vi "cRIO IO Simulation.vi"() -> ()   [LabVIEW 2024, in "cRIO1.lvlib"]
doc: "Simulates a PID controller."
uses:
  cRIO1.lvlib
  PID - Data.ctl
panel:
  out "error out":errorcluster
  out "output chart":dbl(graph)
  in  "Stop":bool
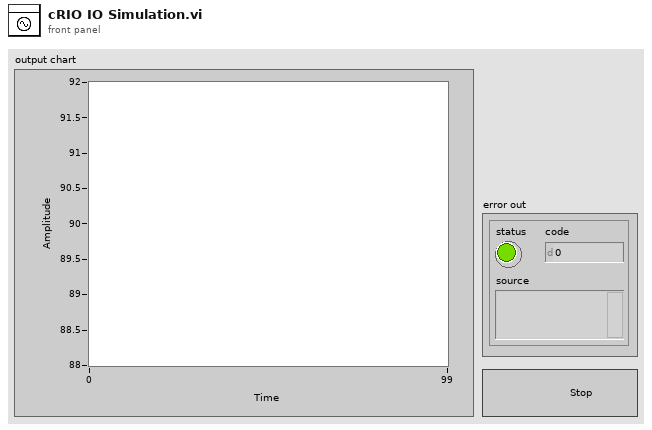
[diagram p1: front panel]
types:
  T1 = typedef "cRIO1.lvlib/PID - Data.ctl" = cluster{"P":dbl, "I":dbl, "D":dbl, "Last Error":dbl, "Total Error":dbl}
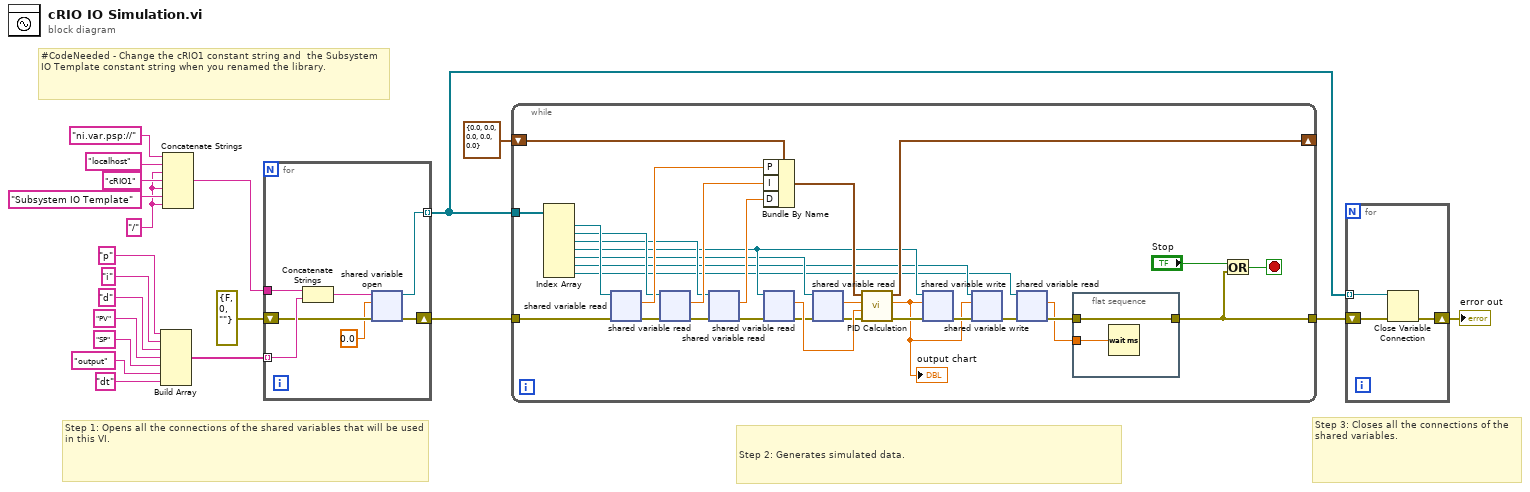
[diagram p0: block diagram]
diagram:
  w3 = "/" ("string")
  # "Step 3: Closes all the connections of the shared variables."
  # "Step 2: Generates simulated data."
  # "#CodeNeeded - Change the cRIO1 constant string and  the Subsystem IO Template constant string when you renamed the library."
  # "Step 1: Opens all the connections of the shared variables that will be used in this VI."
  n1 = Build Array("p" ("string"), "i" ("string"), "d" ("string"), "PV" ("string"), "SP" ("string"), "output" ("string"), "dt" ("string")) -> (w13:string[])
  n2 = Concatenate Strings("ni.var.psp://" ("string"), "localhost" ("string"), w3, "cRIO1" ("string"), w3, "Subsystem IO Template" ("string"), w3) -> (w8:string)
  n3 = for {
    tunnel: w8 -> [w27]
    tunnel: w13 -> [w26] mode=indexing
    tunnel: [w23] -> w2 mode=indexing
    shift-right: [w24] -> w11
    shift-left: errorcluster {"status"=FALSE, "code"=0, "source"=""} ("Error Out") -> [w22]
    n4 = Concatenate Strings(w27, w26) -> (w25:string)
    n5 = shared-variable-open ("Open Variable Connection")(w25, w22, 0.0 ("milliseconds to wait")) -> (w23:refnum<k21>, w24:errorcluster)  [unwired: 1 in]
  }
  n6 = while {
    shift-right: [w58] -> _
    shift-left: T1 {"P"=0.0, "I"=0.0, "D"=0.0, "Last Error"=0.0, "Total Error"=0.0} ("PID") -> [w57]
    tunnel: w11 -> [w53]
    tunnel: [w38] -> w10
    tunnel: w2 -> [w37]
    stop <- w54 stop-if-true
    n7 = Index Array(array=w37) -> (element #1=w36:refnum<k21>, element #2=w35:refnum<k21>, element #3=w34:refnum<k21>, element #4=w33:refnum<k21>, element #5=w32:refnum<k21>, element #6=w31:refnum<k21>, element #7=w28:refnum<k21>)  [unwired: 7 in]
    n8 = shared-variable-read ("Read Variable")(w36, w53) -> (w52:errorcluster, w50:dbl)  [unwired: 2 out]
    n9 = shared-variable-read ("Read Variable")(w35, w52) -> (w51:errorcluster, w49:dbl)  [unwired: 2 out]
    n10 = shared-variable-read ("Read Variable")(w34, w51) -> (w47:errorcluster, w48:dbl)  [unwired: 2 out]
    n11 = Bundle By Name(cluster=w57, "P"=w50, "I"=w49, "D"=w48) -> (w56:T1)
    n12 = shared-variable-read ("Read Variable")(w33, w47) -> (w45:errorcluster, w46:dbl)  [unwired: 2 out]
    n13 = shared-variable-read ("Read Variable")(w32, w45) -> (w44:errorcluster, w43:dbl)  [unwired: 2 out]
    n14 = call "PID Calculation.vi"("error in (no error)"=w44, "PV"=w46, "SP"=w43, "PID - Data In"=w56) -> ("error out"=w42:errorcluster, "output"=w40:dbl, "PID - Data Out"=w58:T1)  [unwired: 5 in]
    "output chart" <- w40
    n15 = shared-variable-write ("Write Variable")(w33, w42, w40) -> (w41:errorcluster)  [unwired: 1 out]
    n16 = shared-variable-write ("Write Variable")(w31, w41, w40) -> (w39:errorcluster)  [unwired: 1 out]
    n17 = shared-variable-read(w28, w39) -> (w30:errorcluster, w29:dbl)  [unwired: 2 out]
    n18 = flat-sequence {
      tunnel: w30 -> [w60]
      tunnel: [w60] -> w38
      tunnel: w29 -> [w59]
      frame #0 {
        n19 = Wait (ms)(milliseconds to wait=w59) -> ()  [unwired: 1 out]
      }
    }
    n20 = Or(x="Stop", y=w38) -> (x .or. y?=w54:bool)
  }
  n21 = for {
    tunnel: w2 -> [w63] mode=indexing
    shift-right: [w61] -> w9
    shift-left: w10 -> [w62]
    n22 = Close Variable Connection(8:w62, 11:w63) -> (0:w61:errorcluster)
  }
  "error out" <- w9
